vi "testVisaCommunication.vi"() -> ()   [LabVIEW 2015]
uses:
  Tektronix AFG 3000 Series/Tektronix AFG 3000 Series.lvlib
panel:
  in  "turn off readind":bool
  out "read buffer":string
  in  "write buffer":string
  out "VISA resource name out":refnum<visa-resource-name>
  out "error out":errorcluster
  in  "error in (no error)":errorcluster
  in  "VISA resource name 2":refnum<visa-resource-name>
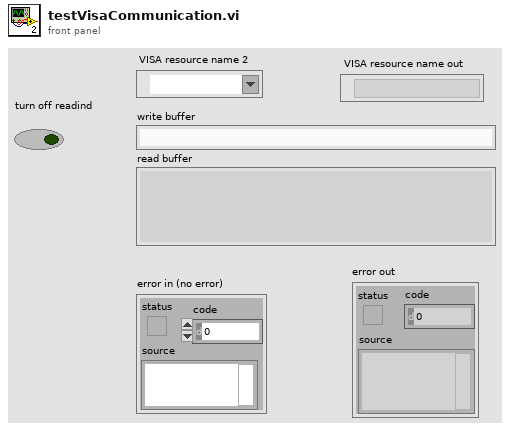
[diagram p1: front panel]
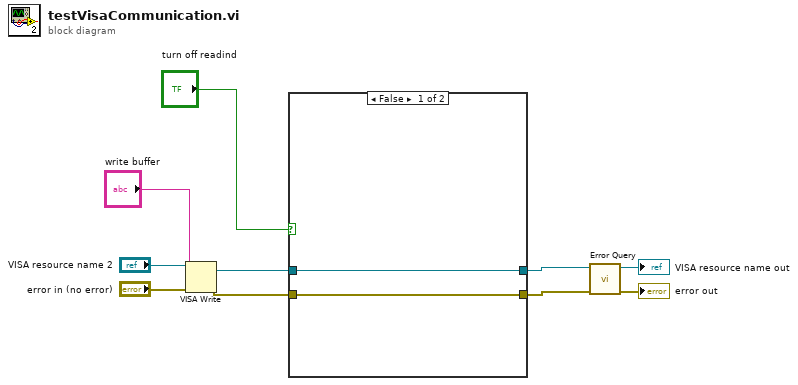
[diagram p0: block diagram]
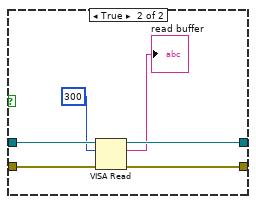
[diagram p2: hidden frame]
diagram:
  n1 = VISA Write(VISA resource name="VISA resource name 2", write buffer="write buffer", error in (no error)="error in (no error)") -> (VISA resource name out=w3:refnum<visa-resource-name>, error out=w5:errorcluster)  [unwired: 1 out]
  n2 = case shown="False" "turn off readind" {
    tunnel: w5 -> [w11 w18]
    tunnel: [w11 w17] -> w4
    tunnel: w3 -> [w12 w16]
    tunnel: [w12 w15] -> w2
    frame False {
    }
    frame True {
      n3 = VISA Read(VISA resource name=w16, byte count=u32 300, error in (no error)=w18) -> (VISA resource name out=w15:refnum<visa-resource-name>, read buffer=→"read buffer":string, error out=w17:errorcluster)  [unwired: 1 out]
    }
  }
  n4 = call "Error Query.vi"("error in (no error)"=w4, "VISA resource name"=w2) -> ("error out"=→"error out":errorcluster, "VISA resource name out"=→"VISA resource name out":refnum<visa-resource-name>)  [unwired: 6 in, 2 out]
